vi "GEA2 Initialize Multiple Devices.vi"(0 "Source Addresses":u8[](array[numeric]) format="%.0x", 11 "error in":errorcluster) -> (4 "Array of GEA2 References Out":refnum<k24>[](array[refnum]), 8 "Board IDs":string[](array[string]), 15 "error out":errorcluster)   [LabVIEW 2016, in "GEA2_Toolkit.lvlib"]
doc: "This VI uses .NET DLLs to initialize a GEA2 connection over USB to multiple devices. The output is an array of references to the newly opened GEA2 connections."
uses:
  library/GEA2_Toolkit.lvlib
  C:/Technology Lab/NI-2010/Trunk/Utility/LabVIEW GEA2 Toolkit v1.0.0.0/Appliance.NET/GeaCommunication.dll
  Appliance.NET/GeaCommunication.dll
  C:/Technology Lab/NI-2010/Trunk/Utility/LabVIEW GEA2 Toolkit v1.0.0.0/Appliance.NET/GeaCommunication.Usb.dll
  Appliance.NET/GeaCommunication.Usb.dll
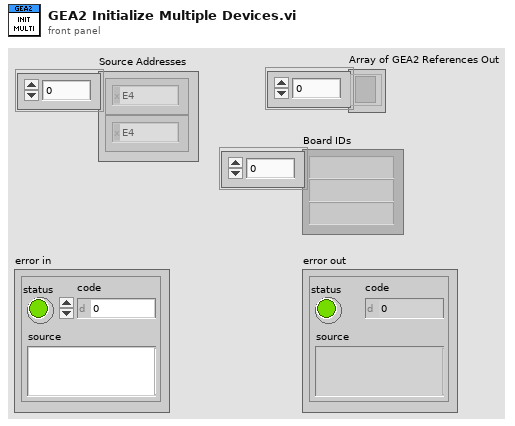
[diagram p1: front panel]
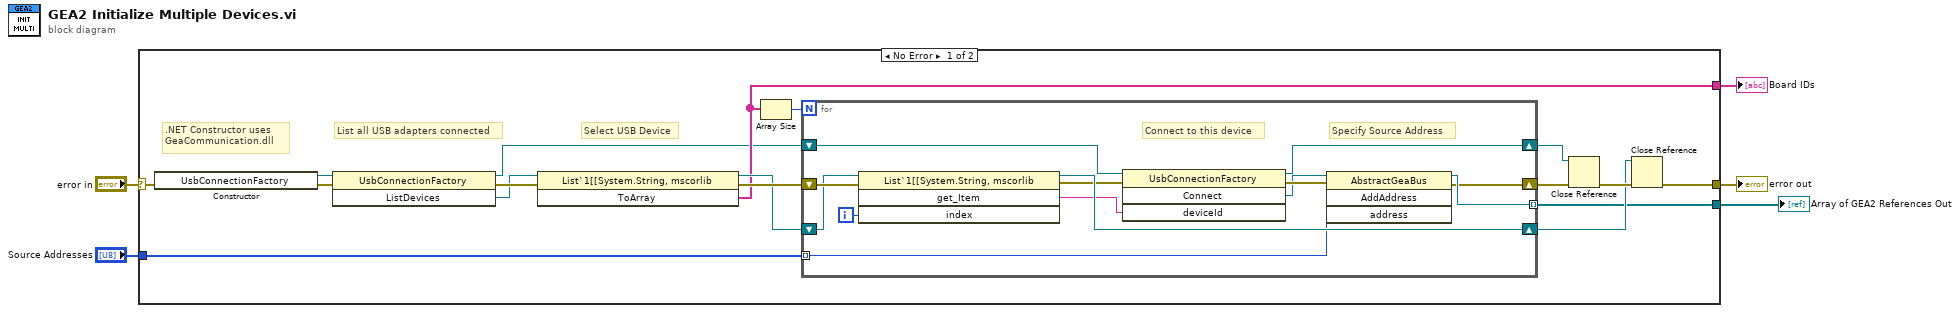
[diagram p0: block diagram]
diagram:
  n1 = case shown="No Error" "error in" {
    selector: "error in" -> [w20 w36]
    tunnel: [w9 w36] -> w5
    tunnel: [w7 _] -> w1
    tunnel: "Source Addresses" -> [w15 _]
    tunnel: [w13 _] -> w2
    frame No Error {
      # "Select USB Device"
      # "List all USB adapters connected"
      # ".NET Constructor uses\nGeaCommunication.dll"
      n2 = constructor class="UsbConnectionFactory"(error in=w20) -> (reference out=w18:refnum<k24>, error out=w19:errorcluster)  [unwired: 2 in, 1 out]
      n3 = invoke class="UsbConnectionFactory" method="ListDevices"(reference=w18, error in=w19) -> (reference out=w6:refnum<k24>, error out=w22:errorcluster, "ListDevices"=w21:refnum<k24>)  [unwired: 1 in]
      n4 = invoke class="List`1[[System.String, mscorlib" method="ToArray"(reference=w21, error in=w22) -> (reference out=w16:refnum<k24>, error out=w17:errorcluster, "ToArray"=w13:string[])  [unwired: 1 in]
      n5 = Array Size(array=w13) -> (size(s)=w14:i32)
      n6 = for {
        N: w14 -> [_]
        tunnel: [w35] -> w7 mode=indexing
        shift-right: [w24] -> w11
        shift-left: w6 -> [w28]
        shift-right: [w30] -> w12
        shift-left: w17 -> [w34]
        shift-right: [w31] -> w8
        shift-left: w16 -> [w33]
        tunnel: w15 -> [w29] mode=indexing
        i -> [w32]
        # "Specify Source Address"
        # "Connect to this device"
        n7 = invoke class="List`1[[System.String, mscorlib" method="get_Item"(reference=w33, error in=w34, "index"=w32) -> (reference out=w31:refnum<k24>, error out=w27:errorcluster, "get_Item"=w23:string)  [unwired: 1 in, 1 out]
        n8 = invoke class="UsbConnectionFactory" method="Connect"(reference=w28, error in=w27, "deviceId"=w23) -> (reference out=w24:refnum<k24>, error out=w26:errorcluster, "Connect"=w25:refnum<k24>)  [unwired: 1 in, 1 out]
        n9 = invoke class="AbstractGeaBus" method="AddAddress"(reference=w25, error in=w26, "address"=w29) -> (reference out=w35:refnum<k24>, error out=w30:errorcluster)  [unwired: 1 in, 2 out]
      }
      n10 = Close Reference(reference=w11, error in (no error)=w12) -> (error out=w10:errorcluster)
      n11 = Close Reference(reference=w8, error in (no error)=w10) -> (error out=w9:errorcluster)
    }
    frame Error {
    }
  }
  "error out" <- w5
  "Board IDs" <- w2
  "Array of GEA2 References Out" <- w1
